vi "Send Add Sink.vi"(8 "error in (no error)":errorcluster, 10 "Log Sink":refnum<class "Log Sink.lvclass">, 11 "LoggerReference in":refnum<class "LoggerReference.lvclass">) -> (0 "Error Out":errorcluster, 2 "Log Sink Reference":refnum<data-value>, 3 "LoggerReference out":refnum<class "LoggerReference.lvclass">)   [LabVIEW 2017, in "Composed Log.lvlib" / "LoggerReference.lvclass"]
uses:
  <vilib>/gpm_packages/@cs/event-logger/Source/Composed Log/LoggerReference/LoggerReference.lvclass
  <vilib>/gpm_packages/@cs/event-logger/Source/Composed Log/Log Sink/Log Sink.lvclass
  <vilib>/gpm_packages/@cs/event-logger/Source/Composed Log/LoggerReference/LoggerReference.lvclass/LoggerReference.ctl
  <vilib>/gpm_packages/@cs/event-logger/Source/Composed Log/Types/MessageCluster.ctl
  <vilib>/gpm_packages/@cs/event-logger/Source/Composed Log/Composed Log.lvlib
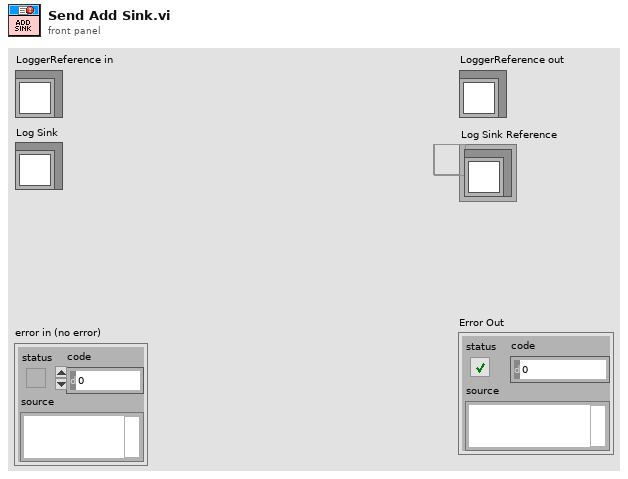
[diagram p1: front panel]
types:
  T1 = typedef "Composed Log.lvlib/MessageCluster.ctl" = cluster{"Message":string, "Data":variant}
  T2 = cluster{"Log Sink":refnum<class "Log Sink.lvclass">, "queue out":refnum<queue>, "queue out":refnum<queue>}
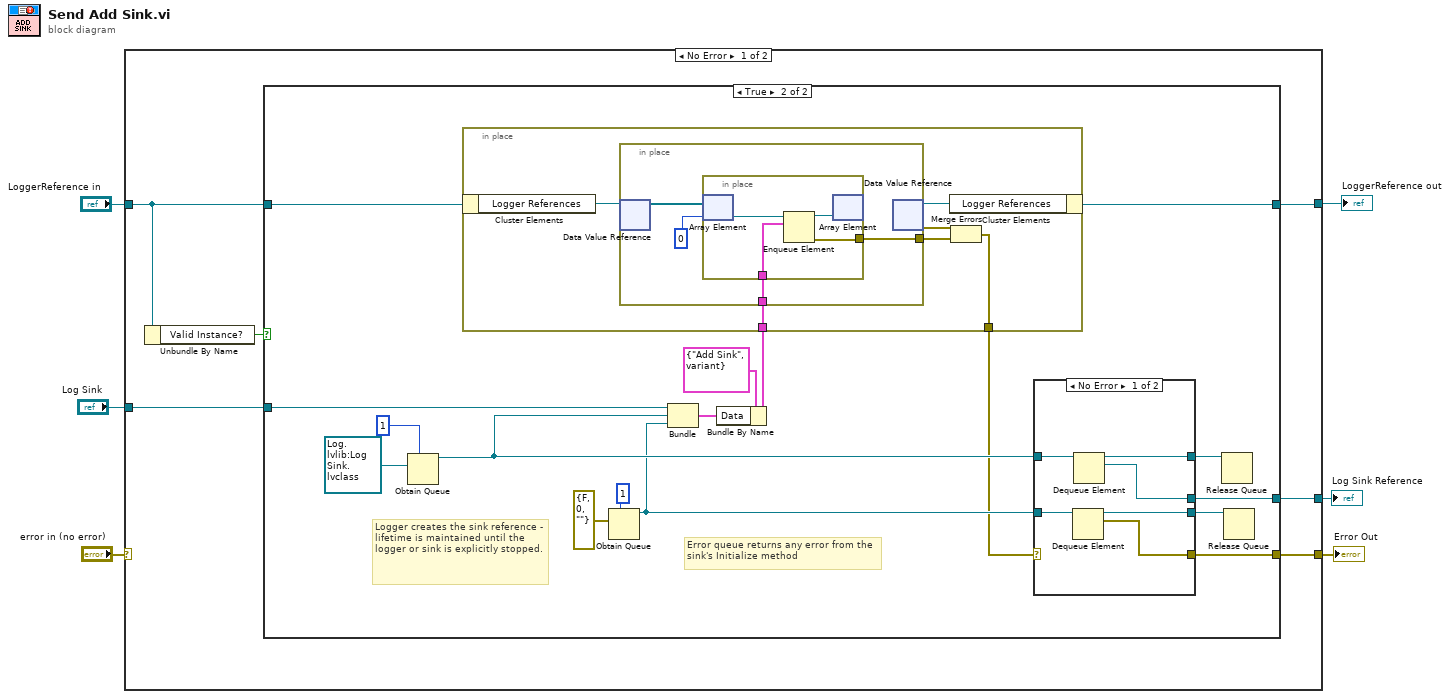
[diagram p0: block diagram]
diagram:
  n1 = case shown="No Error" "error in (no error)" {
    selector: "error in (no error)" -> [_ w54]
    tunnel: "Log Sink" -> [w12 _]
    tunnel: [w11 _] -> w1
    tunnel: "LoggerReference in" -> [w8 w55]
    tunnel: [w7 w55] -> w4
    tunnel: [w10 w54] -> w2
    frame No Error {
      n2 = Unbundle By Name(w8) -> ("Valid Instance?"=w9:bool)
      n3 = case shown="True" w9 {
        tunnel: w12 -> [_ w22]
        tunnel: [_ w21] -> w11
        tunnel: [_ w20] -> w10
        tunnel: w8 -> [w13 w18]
        tunnel: [w13 w17] -> w7
        frame False {
        }
        frame True {
          # "Error queue returns any error from the sink's Initialize method"
          # "Logger creates the sink reference - lifetime is maintained until the logger or sink is explicitly stopped."
          n4 = Obtain Queue(max queue size (-1, unlimited)=1, element data type=refnum<data-value> refnum ("Log Sink Reference")) -> (queue out=w24:refnum<queue>)  [unwired: 3 in, 2 out]
          n5 = Obtain Queue(max queue size (-1, unlimited)=1, element data type=errorcluster {"status"=FALSE, "code"=0, "source"=""} ("error in (no error)")) -> (queue out=w23:refnum<queue>)  [unwired: 3 in, 2 out]
          n6 = Bundle("Log Sink"=w22, "queue out"=w24, "queue out"=w23) -> (w14:T2)  [unwired: 1 in]
          n7 = Bundle By Name(cluster=T1 {"Message"="Add Sink", "Data"=variant} ("Cluster"), "Data"=w14) -> (w16:T1)
          n8 = in-place {
            in-place-border: [w32] -> w19
            in-place-border: w16 -> [w31]
            n9 = in-place-cluster #1(w18) -> ("Logger References"=w36:refnum<data-value>)
            n10 = in-place {
              in-place-border: [w38] -> w33
              in-place-border: w31 -> [w37]
              n11 = in-place-dvr #2(w36) -> (w40:refnum<queue>[])  [unwired: 1 out]
              n12 = in-place {
                in-place-border: [w42] -> w38
                in-place-border: w37 -> [w41]
                n13 = in-place-array #3(w40, 0) -> (w44:refnum<queue>)
                n14 = Enqueue Element(queue=w44, element=w41) -> (queue out=w43:refnum<queue>, error out=w42:errorcluster)  [unwired: 2 in, 1 out]
                n15 = in-place-array #3(w43) -> ()  [unwired: 2 out]
              }
              n16 = in-place-dvr #2() -> (w35:refnum<data-value>, w34:errorcluster)  [unwired: 1 in]
            }
            n17 = in-place-cluster #1("Logger References"=w35) -> (w17:refnum<class "LoggerReference.lvclass">)
            n18 = Merge Errors(w34, w33) -> (w32:errorcluster)
          }
          n19 = case shown="No Error" w19 {
            selector: w19 -> [_ w51]
            tunnel: w24 -> [w50 w52]
            tunnel: w23 -> [w49 w53]
            tunnel: [w48 _] -> w21
            tunnel: [w47 w52] -> w26
            tunnel: [w46 w53] -> w25
            tunnel: [w45 w51] -> w20
            frame No Error {
              n20 = Dequeue Element(queue=w49) -> (queue out=w46:refnum<queue>, element=w45:errorcluster)  [unwired: 2 in, 2 out]
              n21 = Dequeue Element(queue=w50) -> (queue out=w47:refnum<queue>, element=w48:refnum<data-value>)  [unwired: 2 in, 2 out]
            }
            frame Error {
            }
          }
          n22 = Release Queue(queue=w26) -> ()  [unwired: 2 in, 3 out]
          n23 = Release Queue(queue=w25) -> ()  [unwired: 2 in, 3 out]
        }
      }
    }
    frame Error {
    }
  }
  "LoggerReference out" <- w4
  "Error Out" <- w2
  "Log Sink Reference" <- w1
